vi "Agilent SNA Trigger and Fetch Measurement.vi"(6 "Channel":i8=1 min=1 max=99 step=1, 7 "Agilent SNA & SWP":T1, 8 "error in (no error)":errorcluster, 10 "Timout, ms (10000)":u32=10000, 11 "VISA Resource Names":T2) -> (0 "error out":errorcluster, 3 "dup VISA Resource Names":T2)   [LabVIEW 2011]
doc: "Takes a SING sweep and returns the magnitude in dB of the requested data"
uses:
  TypeDefs/Agilent SNA VISA.ctl
  TypeDefs/Agilent SNA Instrument Info.ctl
  TypeDefs/Agilent SNA Trigger Mode.ctl
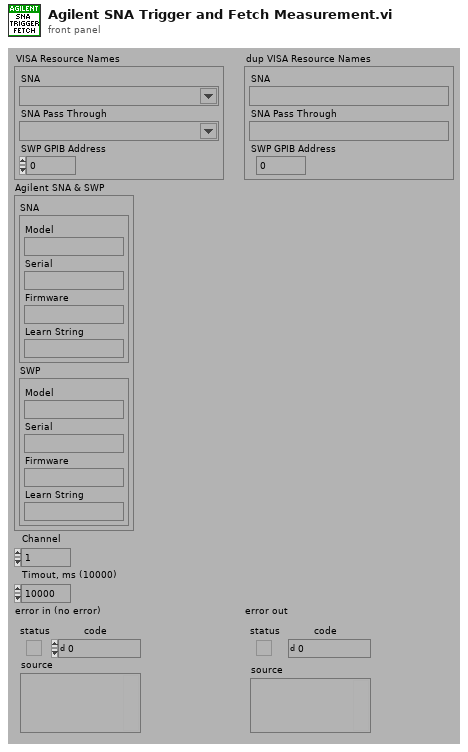
[diagram p1: front panel]
types:
  T1 = typedef "Agilent SNA Instrument Info.ctl" = cluster{"SNA":cluster{"Model":string, "Serial":string, "Firmware":string, "Learn String":string}, "SWP":cluster{"Model":string, "Serial":string, "Firmware":string, "Learn String":string}}
  T2 = typedef "Agilent SNA VISA.ctl" = cluster{"SNA":refnum<visa-resource-name>, "SNA Pass Through":refnum<visa-resource-name>, "SWP GPIB Address":i32}
  T3 = typedef "Agilent SNA Trigger Mode.ctl" = enum16{"Continuous", "Hold", "Single"}
  T4 = typedef "Agilent SNA Model.ctl" = enum16{"Not Supported", "8757X"}
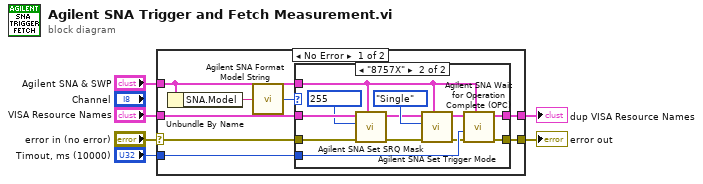
[diagram p0: block diagram]
diagram:
  n1 = case shown="No Error" "error in (no error)" {
    selector: "error in (no error)" -> [w13 w30]
    tunnel: "VISA Resource Names" -> [w14 w29]
    tunnel: "Timout, ms (10000)" -> [w12 _]
    tunnel: [w11 w30] -> w3
    tunnel: [w10 w29] -> w4
    tunnel: "Agilent SNA & SWP" -> [w8 _]
    frame No Error {
      n2 = Unbundle By Name(w8) -> ("SNA.Model"=w7:string)
      n3 = call "Agilent SNA Format Model String.vi"("Model String"=w7) -> ("Model"=w9:T4)
      n4 = case shown="\"8757X\"" w9 {
        tunnel: w14 -> [w16 w23]
        tunnel: w13 -> [w15 w19]
        tunnel: w12 -> [_ w27]
        tunnel: [w15 w26] -> w11
        tunnel: [w16 w25] -> w10
        tunnel: w8 -> [_ w22]
        frame "Not Supported" {
        }
        frame "8757X" {
          n5 = call "Agilent SNA Set SRQ Mask.vi"("Agilent SNA & SWP"=w22, "error in (no error)"=w19, "SRQ Mask"=u8 255, "VISA Resource Names"=w23) -> ("error out"=w20:errorcluster, "dup VISA Resource Names"=w21:T2)  [unwired: 1 in, 5 out]
          n6 = call "Agilent SNA Set Trigger Mode.vi"("Agilent SNA & SWP"=w22, "error in (no error)"=w20, "Trigger Mode"=Agilent_SNA_Trigger_Mode."Single", "VISA Resource Names"=w21) -> ("error out"=w17:errorcluster, "dup VISA Resource Names"=w28:T2)  [unwired: 1 in, 5 out]
          n7 = call "Agilent SNA Wait for Operation Complete (OPC).vi"("Agilent SNA & SWP"=w22, "error in (no error)"=w17, "Timeout, ms (10000)"=w27, "VISA Resource Names"=w28) -> ("error out"=w26:errorcluster, "dup VISA Resource Names"=w25:T2)  [unwired: 6 out]
        }
      }
    }
    frame Error {
      # "Incoming Error....do nothing."
    }
  }
  "dup VISA Resource Names" <- w4
  "error out" <- w3
